vi "Custom Swerve Drive.vi"(3 "Motor Extremes":T9, 4 "Right Direction Motor Refnum":T2={"DeviceStatus"={"status"=FALSE, "code"=0, "source"=""}, "Type"=enum."PWM", "PWM"={"Digital Module"=enum."Digital Module 1", "PWM Channel"=enum."Invalid", "DeadBand"={"Name"="", "maxPositivePwm"=0, "minPositivePwm"=0, "centerPwm"=0, "maxNegativePwm"=0, "minNegativePwm"=0, "angularRange"=0}}, "CAN"={"Device Number"=0, "Control Mode"=enum."Percent VBus", "Semaphore"=refnum, "Max Vout"=12.0}, "Invert"=FALSE, "TransformRef"=refnum, "InvTransformRef"=refnum}, 5 "Left Direction Motor Refnum":T2={"DeviceStatus"={"status"=FALSE, "code"=0, "source"=""}, "Type"=enum."PWM", "PWM"={"Digital Module"=enum."Digital Module 1", "PWM Channel"=enum."Invalid", "DeadBand"={"Name"="", "maxPositivePwm"=0, "minPositivePwm"=0, "centerPwm"=0, "maxNegativePwm"=0, "minNegativePwm"=0, "angularRange"=0}}, "CAN"={"Device Number"=0, "Control Mode"=enum."Percent VBus", "Semaphore"=refnum, "Max Vout"=12.0}, "Invert"=FALSE, "TransformRef"=refnum, "InvTransformRef"=refnum}, 6 "Robot Drive Refnum":T1={"DevStatus"={"status"=FALSE, "code"=0, "source"=""}, "Motors[]"=[], "Square Inputs"=FALSE, "Max Output"=1.0, "Isochronous"=FALSE}, 7 "Xbox Refnum":T10) -> (1 "Motor Values":dbl[](array[numeric]))   [LabVIEW 2013]
doc: "Utilizes WPI Robotics Library to create a dual-motor swerve drive coupled with an XBox controller."
uses:
  <vilib>/Rock Robotics/WPI/MotorControl/WPI_MotorControlDeviceRef.ctl
  <vilib>/Rock Robotics/SystemInterfaces/Typedef/FPGA_TypedefDigitalModule.ctl
  <vilib>/Rock Robotics/SystemInterfaces/DIO/FPGA_DIOPWMChannel.ctl
  <vilib>/Rock Robotics/WPI/PWM/WPI_PWMDeadband.ctl
  <vilib>/Rock Robotics/WPI/CAN/Jaguar/SubVIs/WPI_CANJaguar_ControlMode.ctl
  <vilib>/Rock Robotics/WPI/PWM/WPI_PWMTransform_ConPane.ctl
  <vilib>/Rock Robotics/WPI/Joystick/WPI_JoystickDevRef.ctl
  <vilib>/Rock Robotics/WPI/Joystick/WPI_JoystickDeviceEnum.ctl
  <vilib>/Rock Robotics/WPI/RobotDrive/WPI_RobotDriveDevRef.ctl
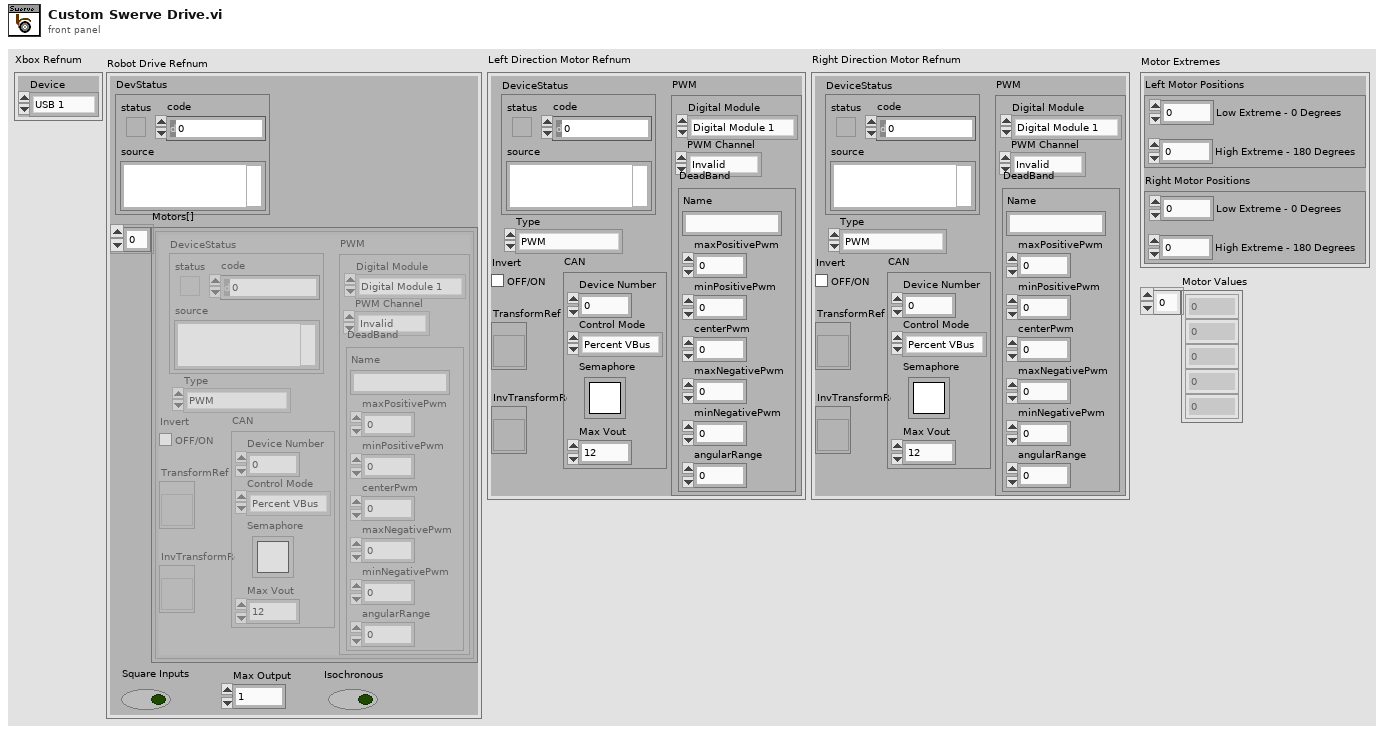
[diagram p1: front panel]
types:
  T1 = typedef "WPI_RobotDriveDevRef.ctl" = cluster{"DevStatus":errorcluster, "Motors[]":T2[], "Square Inputs":bool, "Max Output":dbl, "Isochronous":bool}
  T2 = typedef "WPI_MotorControlDeviceRef.ctl" = cluster{"DeviceStatus":errorcluster, "Type":enum16{"PWM", "CAN"}, "PWM":cluster{"Digital Module":T3, "PWM Channel":T4, "DeadBand":T5}, "CAN":cluster{"Device Number":u8, "Control Mode":T6, "Semaphore":T7, "Max Vout":dbl}, "Invert":bool, "TransformRef":T8, "InvTransformRef":T8}
  T3 = typedef "FPGA_TypedefDigitalModule.ctl" = enum16{"Digital Module 1", "Digital Module 2"}
  T4 = typedef "FPGA_DIOPWMChannel.ctl" = enum8{"PWM 1", "PWM 2", "PWM 3", "PWM 4", "PWM 5", "PWM 6", "PWM 7", "PWM 8", "PWM 9", "PWM 10", "Invalid"}
  T5 = typedef "WPI_PWMDeadband.ctl" = cluster{"Name":string, "maxPositivePwm":i32, "minPositivePwm":i32, "centerPwm":i32, "maxNegativePwm":i32, "minNegativePwm":i32, "angularRange":u16}
  T6 = typedef "WPI_CANJaguar_ControlMode.ctl" = enum8{"Percent VBus", "Current", "Speed", "Position", "Voltage"}
  T7 = typedef "Semaphore RefNum" = refnum<k1>
  T8 = typedef "WPI_PWMTransform_ConPane.ctl" = refnum<vi>
  T9 = cluster{"Left Motor Positions":cluster{"Low Extreme - 0 Degrees":dbl, "High Extreme - 180 Degrees":dbl}, "Right Motor Positions":cluster{"Low Extreme - 0 Degrees":dbl, "High Extreme - 180 Degrees":dbl}}
  T10 = typedef "WPI_JoystickDevRef.ctl" = cluster{"Device":T11}
  T11 = typedef "WPI_JoystickDeviceEnum.ctl" = enum16{"USB 1", "USB 2", "USB 3", "USB 4", "Kinect 1", "Kinect 2"}
  T12 = cluster{"axis 1 (x)":dbl, "axis 2 (y)":dbl, "axis 3 (throttle)":dbl, "axis 4":dbl, "axis 5":dbl, "axis 6":dbl}
  T13 = cluster{"Low Extreme - 0 Degrees":dbl, "High Extreme - 180 Degrees":dbl}
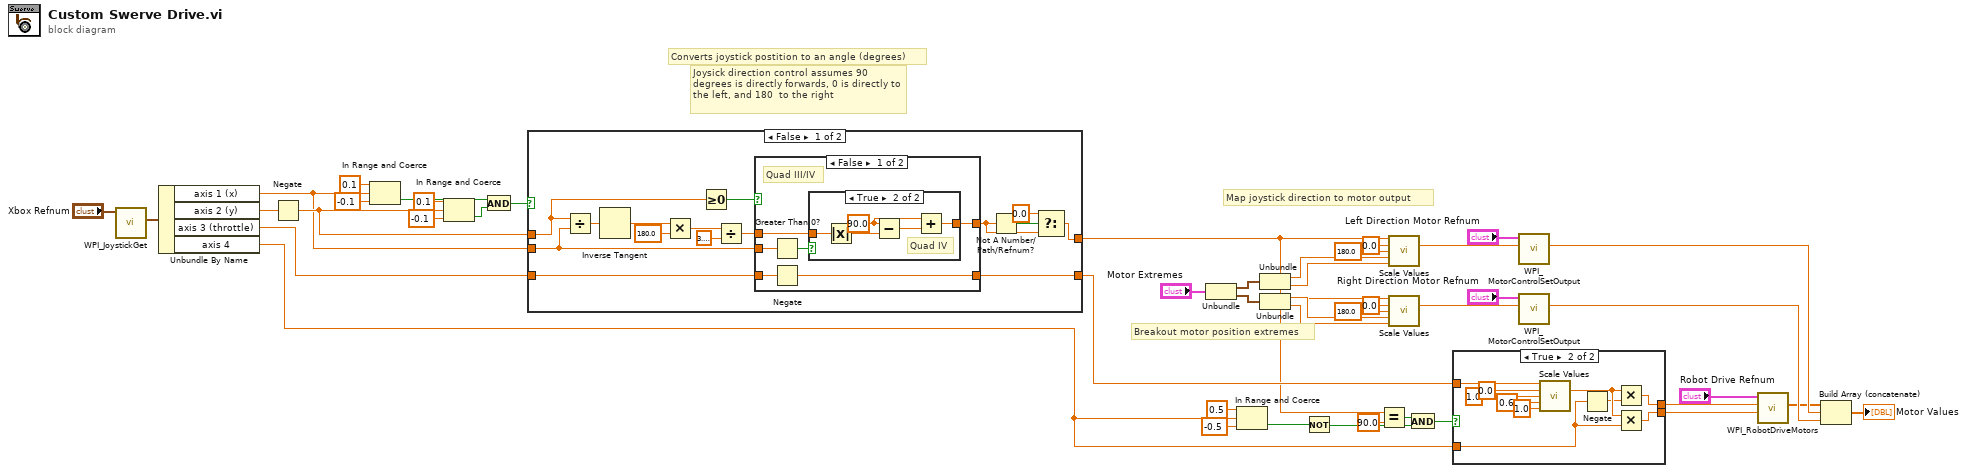
[diagram p0: block diagram]
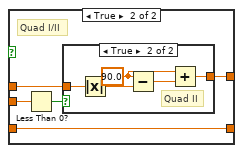
[diagram p3: hidden frame]
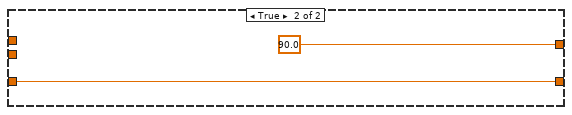
[diagram p5: hidden frame]
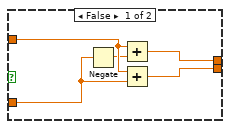
[diagram p6: hidden frame]
diagram:
  # "Joysick direction control assumes 90 degrees is directly forwards, 0 is directly to the left, and 180  to the right"
  # "Breakout motor position extremes"
  # "Converts joystick postition to an angle (degrees)"
  # "Map joystick direction to motor output"
  n1 = call <vilib>:"WPI_JoystickGet.vi"("JoystickDevRef"="Xbox Refnum") -> ("Axes"=w43:T12)  [unwired: 4 in, 2 out]
  n2 = Unbundle By Name(w43) -> ("axis 1 (x)"=w4:dbl, "axis 2 (y)"=w5:dbl, "axis 3 (throttle)"=w3:dbl, "axis 4"=w18:dbl)
  n3 = Negate(x=w5) -> (-x=w6:dbl)
  n4 = In Range and Coerce(upper limit=0.1, x=w4, lower limit=-0.1) -> (In Range?=w8:bool)  [unwired: 1 out]
  n5 = In Range and Coerce(upper limit=0.1, x=w6, lower limit=-0.1) -> (In Range?=w9:bool)  [unwired: 1 out]
  n6 = And(x=w8, y=w9) -> (x .and. y?=w7:bool)
  n7 = case shown="False" w7 {
    tunnel: w4 -> [w56 _]
    tunnel: w6 -> [w55 _]
    tunnel: w3 -> [w57 w85]
    tunnel: [w46 90.0] -> w1
    tunnel: [w53 w85] -> w2
    frame False {
      n8 = Divide(x=w55, y=w56) -> (x/y=w60:dbl)
      n9 = Inverse Tangent(1:w60) -> (0:w58:dbl)
      n10 = Multiply(x=w58, y=180.0) -> (x*y=w52:dbl)
      n11 = Greater Or Equal To 0?(x=w55) -> (x >= 0?=w54:bool)
      n12 = Divide(x=w52, y=3.141592653589793) -> (x/y=w51:dbl)
      n13 = case shown="False" w54 {
        tunnel: w57 -> [w63 w73]
        tunnel: w56 -> [w64 w77]
        tunnel: w51 -> [w65 w75]
        tunnel: [w62 w73] -> w53
        tunnel: [w61 w74] -> w47
        frame False {
          # "Quad III/IV"
          n14 = Greater Than 0?(x=w64) -> (x > 0?=w66:bool)
          n15 = Negate(x=w63) -> (-x=w62:dbl)
          n16 = case shown="True" w66 {
            tunnel: w65 -> [w67 w72]
            tunnel: [w67 w68] -> w61
            frame False {
              # "Quad III"
            }
            frame True {
              w69 = 90.0 ("x")
              # "Quad IV"
              n17 = Absolute Value(x=w72) -> (abs(x)=w71:dbl)
              n18 = Subtract(x=w69, y=w71) -> (x-y=w70:dbl)
              n19 = Add(x=w69, y=w70) -> (x+y=w68:dbl)
            }
          }
        }
        frame True {
          # "Quad I/II"
          n20 = Less Than 0?(x=w77) -> (x < 0?=w76:bool)
          n21 = case shown="True" w76 {
            tunnel: w75 -> [w78 w83]
            tunnel: [w78 w79] -> w74
            frame False {
              # "Quad I"
            }
            frame True {
              w80 = 90.0 ("x")
              # "Quad II"
              n22 = Absolute Value(x=w83) -> (abs(x)=w82:dbl)
              n23 = Subtract(x=w80, y=w82) -> (x-y=w81:dbl)
              n24 = Add(x=w80, y=w81) -> (x+y=w79:dbl)
            }
          }
        }
      }
      n25 = Not A Number/Path/Refnum?(number/path/refnum=w47) -> (NaN/Path/Refnum?=w49:bool)
      n26 = Select(t=0.0, s=w49, f=w47) -> (s? t:f=w46:dbl)
    }
    frame True {
    }
  }
  n27 = Unbundle("Motor Extremes") -> ("Left Motor Positions"=w16:T13, "Right Motor Positions"=w15:T13)
  n28 = In Range and Coerce(upper limit=0.5, x=w18, lower limit=-0.5) -> (In Range?=w19:bool)  [unwired: 1 out]
  n29 = Unbundle(w16) -> ("Low Extreme - 0 Degrees"=w38:dbl, "High Extreme - 180 Degrees"=w37:dbl)
  n30 = Unbundle(w15) -> ("Low Extreme - 0 Degrees"=w34:dbl, "High Extreme - 180 Degrees"=w33:dbl)
  n31 = Not(x=w19) -> (.not. x?=w20:bool)
  n32 = Equal?(x=w1, y=90.0) -> (x = y?=w22:bool)
  n33 = call "Scale Values.vi"("input variable"=w1, "input min"=0.0, "input max"=180.0, "output min"=w38, "output max"=w37) -> ("output variable"=w32:dbl)  [unwired: 10 in]
  n34 = call "Scale Values.vi"("input variable"=w1, "input min"=0.0, "input max"=180.0, "output min"=w34, "output max"=w33) -> ("output variable"=w31:dbl)  [unwired: 10 in]
  n35 = And(x=w22, y=w20) -> (x .and. y?=w23:bool)
  n36 = case shown="True" w23 {
    tunnel: w18 -> [w86 w91]
    tunnel: w2 -> [w88 w97]
    tunnel: [w90 w100] -> w25
    tunnel: [w89 w99] -> w24
    frame False {
      n37 = Negate(x=w86) -> (-x=w87:dbl)
      n38 = Add(x=w88, y=w87) -> (x+y=w90:dbl)
      n39 = Add(x=w88, y=w86) -> (x+y=w89:dbl)
    }
    frame True {
      n40 = call "Scale Values.vi"("input variable"=w97, "input min"=0.0, "input max"=1.0, "output min"=0.6, "output max"=1.0) -> ("output variable"=w98:dbl)  [unwired: 10 in]
      n41 = Negate(x=w91) -> (-x=w92:dbl)
      n42 = Multiply(x=w98, y=w92) -> (x*y=w100:dbl)
      n43 = Multiply(x=w98, y=w91) -> (x*y=w99:dbl)
    }
  }
  n44 = call <vilib>:"WPI_MotorControlSetOutput.vi"("Output"=w32, "MotorControlDevRef"="Left Direction Motor Refnum") -> ("Motor Output"=w30:dbl)  [unwired: 7 in, 2 out]
  n45 = call <vilib>:"WPI_MotorControlSetOutput.vi"("Output"=w31, "MotorControlDevRef"="Right Direction Motor Refnum") -> ("Motor Output"=w29:dbl)  [unwired: 7 in, 2 out]
  n46 = call <vilib>:"WPI_RobotDriveMotors.vi"("RightSpeed"=w24, "LeftSpeed"=w25, "RobotDriveDevRef"="Robot Drive Refnum") -> ("Motor Values"=w28:dbl[])  [unwired: 6 in, 2 out]
  n47 = Build Array (concatenate)(w28, w30, w29) -> (→"Motor Values":dbl[])
